vi "Mode3-RAM.vi"() -> (3 "PAARD Super Mode":T5(array[cluster]))   [LabVIEW 2017]
uses:
  Classes/Sequence/SequenceSubvis/TestStep-StepType.ctl
  Classes/Sequence/SequenceSubvis/TestStepTypes.ctl
  Classes/Sequence/SequenceSubvis/RF Direction.ctl
  Classes/Sequence/SequenceSubvis/PolarizationSelect.ctl
  <vilib>/Utility/file.llb/Read Delimited Spreadsheet (DBL).vi
panel:
  in  "Polarization(s)":T1[](array[typedef])=[enum."Horizontal"]
  in  "Probe Vertical Polarization":bool
  in  "Probe Horizontal Polarization":bool
  in  "Probe Tx/Rx":bool
  in  "Data File to Save":path
  in  "Upload TR Module file":path=path "C:/Users/Public/Documents/OU PAARD/mmWave_RF_Scanner/SupportFiles/Mode3example1.csv"
  out "# steps":i32
  out "length, bytes":i32 format="%.3p"
  in  "file path for testing":path=path "Z:/VMShare/OU Scanner/From OU/RodrigoFiles/example3.csv"
  in  "This is the File contents":T2(array[cluster])=[{"X mm"=4.0, "Y mm"=0.0, "File Path"=path ""}, {"X mm"=0.0, "Y mm"=0.0, "File Path"=path ""}, {"X mm"=0.0, "Y mm"=0.0, "File Path"=path ""}, {"X mm"=0.0, "Y mm"=0.0, "File Path"=path ""}, {"X mm"=0.0, "Y mm"=0.0, "File Path"=path ""}, {"X mm"=0.0, "Y mm"=0.0, "File Path"=path ""}, {"X mm"=0.0, "Y mm"=0.0, "File Path"=path ""}, {"X mm"=0.0, "Y mm"=0.0, "File Path"=path ""}, {"X mm"=0.0, "Y mm"=0.0, "File Path"=path ""}, {"X mm"=0.0, "Y mm"=0.0, "File Path"=path ""}, {"X mm"=0.0, "Y mm"=0.0, "File Path"=path ""}, {"X mm"=0.0, "Y mm"=0.0, "File Path"=path ""}, {"X mm"=0.0, "Y mm"=0.0, "File Path"=path ""}, {"X mm"=0.0, "Y mm"=0.0, "File Path"=path ""}, {"X mm"=0.0, "Y mm"=0.0, "File Path"=path ""}, {"X mm"=0.0, "Y mm"=0.0, "File Path"=path ""}, {"X mm"=0.0, "Y mm"=0.0, "File Path"=path ""}, {"X mm"=0.0, "Y mm"=0.0, "File Path"=path ""}, {"X mm"=0.0, "Y mm"=0.0, "File Path"=path ""}, {"X mm"=0.0, "Y mm"=0.0, "File Path"=path ""}, {"X mm"=0.0, "Y mm"=0.0, "File Path"=path ""}, {"X mm"=0.0, "Y mm"=0.0, "File Path"=path ""}, {"X mm"=0.0, "Y mm"=0.0, "File Path"=path ""}, {"X mm"=0.0, "Y mm"=0.0, "File Path"=path ""}, {"X mm"=0.0, "Y mm"=0.0, "File Path"=path ""}, {"X mm"=0.0, "Y mm"=0.0, "File Path"=path ""}, {"X mm"=0.0, "Y mm"=0.0, "File Path"=path ""}, {"X mm"=0.0, "Y mm"=0.0, "File Path"=path ""}, {"X mm"=0.0, "Y mm"=0.0, "File Path"=path ""}, {"X mm"=0.0, "Y mm"=0.0, "File Path"=path ""}, {"X mm"=0.0, "Y mm"=0.0, "File Path"=path ""}, {"X mm"=0.0, "Y mm"=0.0, "File Path"=path ""}, {"X mm"=0.0, "Y mm"=0.0, "File Path"=path ""}, {"X mm"=0.0, "Y mm"=0.0, "File Path"=path ""}, {"X mm"=0.0, "Y mm"=0.0, "File Path"=path ""}, {"X mm"=0.0, "Y mm"=0.0, "File Path"=path ""}, {"X mm"=0.0, "Y mm"=0.0, "File Path"=path ""}, {"X mm"=0.0, "Y mm"=0.0, "File Path"=path ""}, {"X mm"=0.0, "Y mm"=0.0, "File Path"=path ""}, {"X mm"=0.0, "Y mm"=0.0, "File Path"=path ""}, {"X mm"=0.0, "Y mm"=0.0, "File Path"=path ""}, {"X mm"=0.0, "Y mm"=0.0, "File Path"=path ""}, {"X mm"=0.0, "Y mm"=0.0, "File Path"=path ""}, {"X mm"=0.0, "Y mm"=0.0, "File Path"=path ""}, {"X mm"=0.0, "Y mm"=0.0, "File Path"=path ""}, {"X mm"=0.0, "Y mm"=0.0, "File Path"=path ""}, {"X mm"=0.0, "Y mm"=0.0, "File Path"=path ""}, {"X mm"=0.0, "Y mm"=0.0, "File Path"=path ""}, {"X mm"=0.0, "Y mm"=0.0, "File Path"=path ""}, {"X mm"=0.0, "Y mm"=0.0, "File Path"=path ""}, {"X mm"=0.0, "Y mm"=0.0, "File Path"=path ""}, {"X mm"=0.0, "Y mm"=0.0, "File Path"=path ""}, {"X mm"=0.0, "Y mm"=0.0, "File Path"=path ""}, {"X mm"=0.0, "Y mm"=0.0, "File Path"=path ""}, {"X mm"=0.0, "Y mm"=0.0, "File Path"=path ""}, {"X mm"=0.0, "Y mm"=0.0, "File Path"=path ""}, {"X mm"=0.0, "Y mm"=0.0, "File Path"=path ""}, {"X mm"=0.0, "Y mm"=0.0, "File Path"=path ""}, {"X mm"=0.0, "Y mm"=0.0, "File Path"=path ""}, {"X mm"=0.0, "Y mm"=0.0, "File Path"=path ""}, {"X mm"=0.0, "Y mm"=0.0, "File Path"=path ""}, {"X mm"=0.0, "Y mm"=0.0, "File Path"=path ""}, {"X mm"=0.0, "Y mm"=0.0, "File Path"=path ""}, {"X mm"=0.0, "Y mm"=0.0, "File Path"=path ""}, {"X mm"=0.0, "Y mm"=0.0, "File Path"=path "C:/Users/Public/Documents/OU PAARD/mmWave_RF_Scanner/SupportFiles/example1.csv"}]
  in  "Probe Tx/Rx":bool
  in  "Probe H/V":bool
  in  "PAARD Mode 1":T6[](array[typedef])
  in  "UCAR Super Sequence":T6[](array[typedef])
  # "Polarization = Probe Polarization"
  # "UI"
  # "what about a longer test that does both H and V?\n\nRule: only Tx or Rx is allowed."
  # "This file conflicts with the \nwhiteboarded user settings."
  # "THERE MUST BE A FILE FOR EVERY XY."
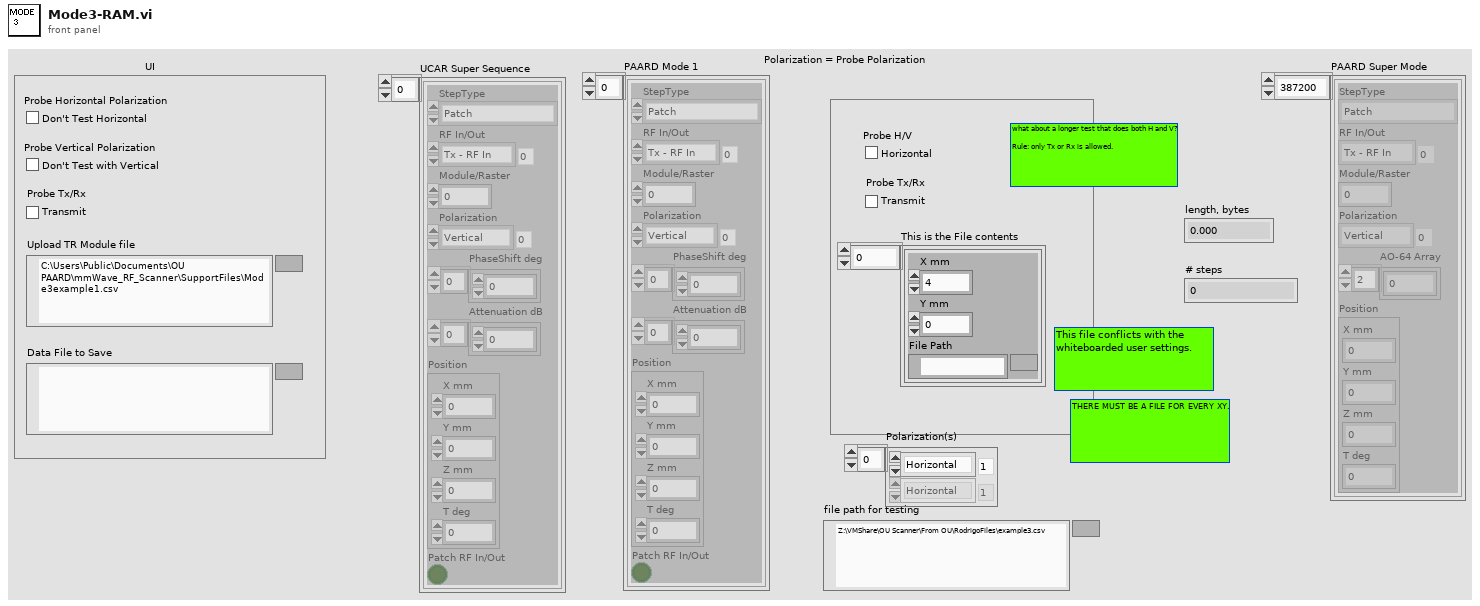
[diagram p1: front panel]
types:
  T1 = typedef "PolarizationSelect.ctl" = enum16{"Vertical", "Horizontal"}
  T2 = cluster{"X mm":dbl, "Y mm":dbl, "File Path":path}[]
  T3 = typedef "TestStepTypes.ctl" = enum16{"Patch", "Motion", "SweepTest", "RasterTest", "Finish", "64ModuleCfg"}
  T4 = typedef "RF Direction.ctl" = enum16{"Tx - RF In", "Rx - RF Out"}
  T5 = cluster{"StepType":T3, "RF In/Out":T4, "Module/Raster":i32, "Polarization":T1, "AO-64 Array":dbl[], "Position":cluster{"X mm":dbl, "Y mm":dbl, "Z mm":dbl, "T deg":dbl}}[]
  T6 = typedef "TestStep-StepType.ctl" = cluster{"StepType":T3, "RF In/Out":T4, "Module/Raster":i32, "Polarization":T1, "PhaseShift deg":dbl[], "Attenuation dB":dbl[], "Position":cluster{"X mm":dbl, "Y mm":dbl, "Z mm":dbl, "T deg":dbl}, "Patch RF In/Out":bool}
  T7 = cluster{"StepType":T3, "RF In/Out":T4, "Module/Raster":i32, "Polarization":T1, "AO-64 Array":dbl[], "Position":cluster{"X mm":dbl, "Y mm":dbl, "Z mm":dbl, "T deg":dbl}}
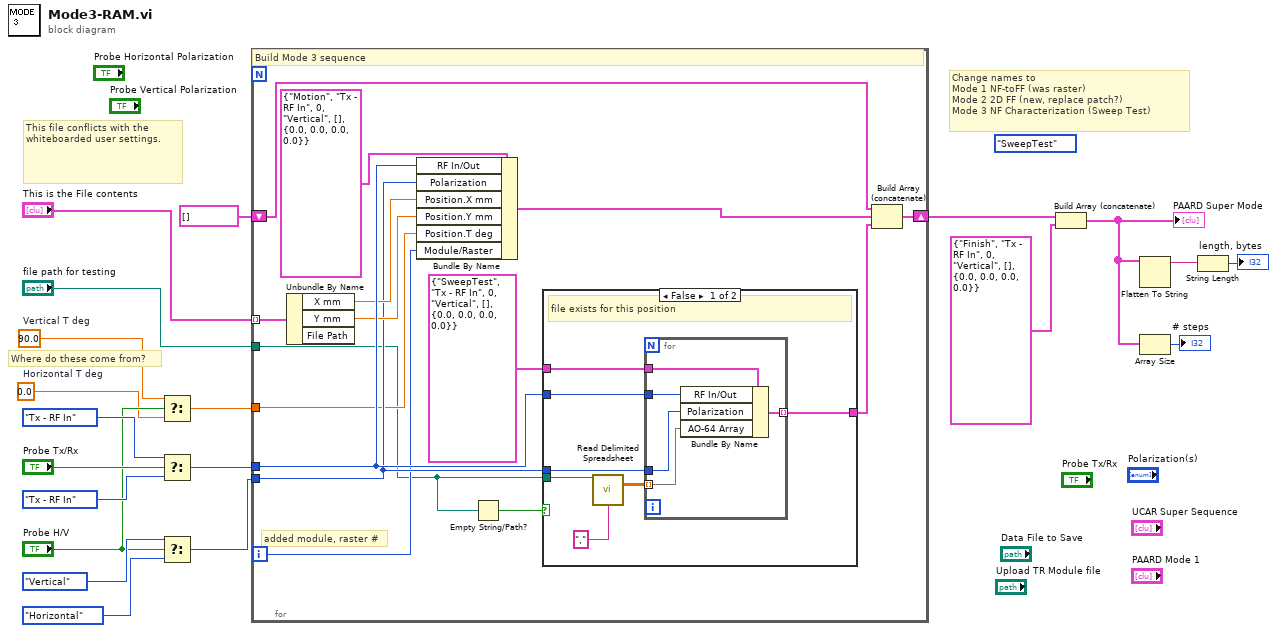
[diagram p0: block diagram]
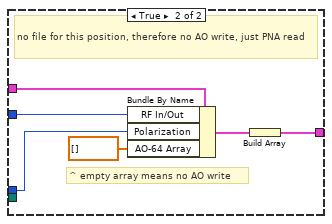
[diagram p2: hidden frame]
diagram:
  (unwired) TestStepTypes."SweepTest" ("StepType")
  w2 = 90.0  # Vertical T deg
  w1 = 0.0  # Horizontal T deg
  # "Change names to \nMode 1 NF-toFF (was raster) \nMode 2 2D FF (new, replace patch?)\nMode 3 NF Characterization (Sweep Test)"
  # "Where do these come from?"
  # "This file conflicts with the \nwhiteboarded user settings."
  n1 = Select(t=w2, s="Probe H/V", f=w1) -> (s? t:f=w10:dbl)
  n2 = Select(t=RF_Direction."Tx - RF In" ("RF In/Out"), s="Probe Tx/Rx", f=RF_Direction."Tx - RF In" ("RF In/Out")) -> (s? t:f=w15:T4)
  n3 = Select(t=PolarizationSelect."Vertical" ("Polarization"), s="Probe H/V", f=PolarizationSelect."Horizontal" ("Polarization")) -> (s? t:f=w14:T1)
  n4 = for {
    tunnel: w15 -> [w33]
    tunnel: w14 -> [w29]
    tunnel: "This is the File contents" -> [w32] mode=indexing
    shift-right: [w28] -> w9
    shift-left: T5 [] -> [w27]
    tunnel: w10 -> [w26]
    tunnel: "file path for testing" -> [w23]
    i -> [w24]
    # "added module, raster #"
    # "Build Mode 3 sequence"
    n5 = Unbundle By Name(w32) -> ("X mm"=w31:dbl, "Y mm"=w30:dbl)  [unwired: 1 out]
    n6 = Bundle By Name(cluster=T7 {"StepType"=enum."Motion", "RF In/Out"=enum."Tx - RF In", "Module/Raster"=0, "Polarization"=enum."Vertical", "AO-64 Array"=[], "Position"={"X mm"=0.0, "Y mm"=0.0, "Z mm"=0.0, "T deg"=0.0}} ("Test"), "RF In/Out"=w33, "Polarization"=w29, "Position.X mm"=w31, "Position.Y mm"=w30, "Position.T deg"=w26, "Module/Raster"=w24) -> (w21:T7)
    n7 = Empty String/Path?(string/path=w23) -> (empty?=w22:bool)
    n8 = case shown="False" w22 {
      tunnel: T7 {"StepType"=enum."SweepTest", "RF In/Out"=enum."Tx - RF In", "Module/Raster"=0, "Polarization"=enum."Vertical", "AO-64 Array"=[], "Position"={"X mm"=0.0, "Y mm"=0.0, "Z mm"=0.0, "T deg"=0.0}} ("Test") -> [w42 w53]
      tunnel: w33 -> [w41 w52]
      tunnel: w29 -> [w39 w51]
      tunnel: [w38 w48] -> w25
      tunnel: w23 -> [w37 _]
      frame False {
        # "file exists for this position"
        n9 = call-poly <vilib>:"Read Delimited Spreadsheet.vi"("file path (dialog if empty)"=w37, "delimiter (\\t)"="," ("delimiter (\\t)")) -> ("all rows"=w40:dbl[][])  [unwired: 8 in, 5 out]
        n10 = for {
          tunnel: w42 -> [w47]
          tunnel: w41 -> [w46]
          tunnel: w40 -> [w45] mode=indexing
          tunnel: w39 -> [w44]
          tunnel: [w43] -> w38 mode=indexing
          n11 = Bundle By Name(cluster=w47, "RF In/Out"=w46, "Polarization"=w44, "AO-64 Array"=w45) -> (w43:T7)
        }
      }
      frame True {
        # "^ empty array means no AO write"
        # "no file for this position, therefore no AO write, just PNA read"
        n12 = Bundle By Name(cluster=w53, "RF In/Out"=w52, "Polarization"=w51, "AO-64 Array"=dbl[] []) -> (w49:T7)
        n13 = Build Array(w49) -> (w48:T5)
      }
    }
    n14 = Build Array (concatenate)(w27, w21, w25) -> (w28:T5)
  }
  n15 = Build Array (concatenate)(w9, T7 {"StepType"=enum."Finish", "RF In/Out"=enum."Tx - RF In", "Module/Raster"=0, "Polarization"=enum."Vertical", "AO-64 Array"=[], "Position"={"X mm"=0.0, "Y mm"=0.0, "Z mm"=0.0, "T deg"=0.0}} ("Test")) -> (w4:T5)
  "PAARD Super Mode" <- w4
  n16 = Flatten To String(anything=w4) -> (data string=w6:string)  [unwired: 3 in, 2 out]
  n17 = Array Size(array=w4) -> (size(s)=→"# steps":i32)
  n18 = String Length(string=w6) -> (length=→"length, bytes":i32)
